vi "颜色常量（汉字）.vi"(11 "颜色":string) -> (3 "颜色常量":u32)   [LabVIEW 2011]
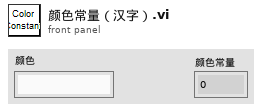
[diagram p1: front panel]
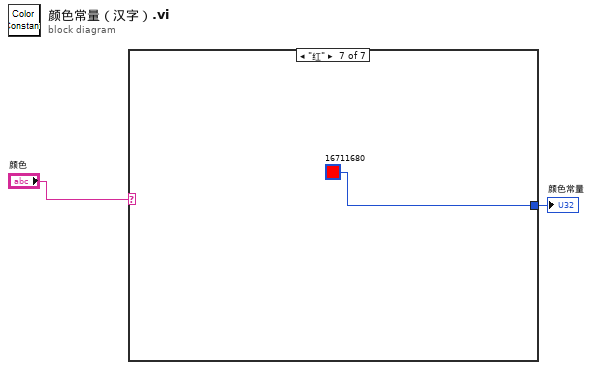
[diagram p0: block diagram]
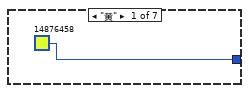
[diagram p2: hidden frame]
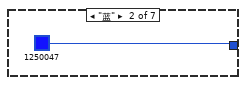
[diagram p3: hidden frame]
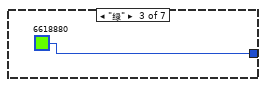
[diagram p4: hidden frame]
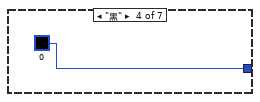
[diagram p5: hidden frame]
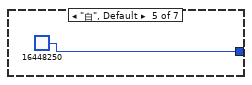
[diagram p6: hidden frame]
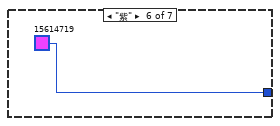
[diagram p7: hidden frame]
diagram:
  n1 = case shown="\"红\"" "颜色" {
    tunnel: [u32 14876458 u32 1250047 u32 6618880 u32 0 u32 16448250 u32 15614719 u32 16711680] -> w1
    frame "黄" {
    }
    frame "蓝" {
    }
    frame "绿" {
    }
    frame "黑" {
    }
    frame "白", Default {
    }
    frame "紫" {
    }
    frame "红" {
    }
  }
  "颜色常量" <- w1
